vi "motorSettings.vi"(8 "error in (no error)":errorcluster, 9 "Velocity (units/s)":dbl=1.0 min=0.0 format="%#.4g", 10 "Acceleration (0 units/s²)":dbl=1.0 min=0.0 format="%#.4g", 11 "VISA Refnum in":refnum<visa-resource-name>) -> (0 "error out":errorcluster, 3 "VISA Refnum out":refnum<visa-resource-name>)   [LabVIEW 2014]
doc: "Newport Motion Controler\n\nSettings \n\nAndré Romero - 2020\nandretec@ifsc.usp.br"
uses:
  <userlib>/Newport ESP301/Newport ESP301.lvlib
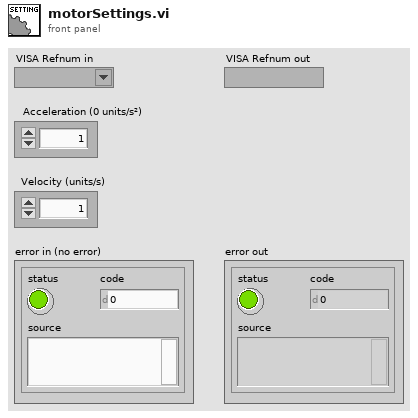
[diagram p1: front panel]
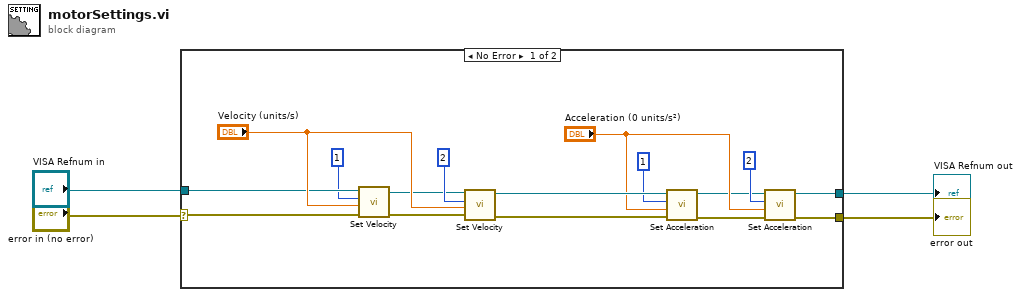
[diagram p0: block diagram]
diagram:
  n1 = case shown="No Error" "error in (no error)" {
    selector: "error in (no error)" -> [w6 w21]
    tunnel: [w20 w22] -> w4
    tunnel: "VISA Refnum in" -> [w11 w22]
    tunnel: [w5 w21] -> w1
    frame No Error {
      n2 = call <userlib>:"Set Velocity.vi"("error in (no error)"=w6, "Velocity (units/s)"="Velocity (units/s)", "Axis (1)"=1, "VISA resource name"=w11) -> ("error out"=w8:errorcluster, "VISA resource name out"=w7:refnum<visa-resource-name>)  [unwired: 2 in]
      n3 = call <userlib>:"Set Velocity.vi"("error in (no error)"=w8, "Velocity (units/s)"="Velocity (units/s)", "Axis (1)"=2, "VISA resource name"=w7) -> ("error out"=w19:errorcluster, "VISA resource name out"=w18:refnum<visa-resource-name>)  [unwired: 2 in]
      n4 = call <userlib>:"Set Acceleration.vi"("error in (no error)"=w19, "Acceleration (0 units/s²)"="Acceleration (0 units/s²)", "Axis (1)"=1, "VISA resource name"=w18) -> ("error out"=w14:errorcluster, "VISA resource name out"=w13:refnum<visa-resource-name>)  [unwired: 2 in]
      n5 = call <userlib>:"Set Acceleration.vi"("error in (no error)"=w14, "Acceleration (0 units/s²)"="Acceleration (0 units/s²)", "Axis (1)"=2, "VISA resource name"=w13) -> ("error out"=w5:errorcluster, "VISA resource name out"=w20:refnum<visa-resource-name>)  [unwired: 2 in]
    }
    frame Error {
    }
  }
  "error out" <- w1
  "VISA Refnum out" <- w4
